vi "CreateEmptyExcelFile.vi"() -> ()   [LabVIEW 2013]
panel:
  in  "# Sheets":i32=1 min=1 step=1
  in  "sheetname":string="Sheet1"
  in  "File Name":path=path "C:/PhaeronGit/LVNPOI/Scratch/test.xls"
  # "LabVIEW implementation of CreateEmptyExcelFile.cs"
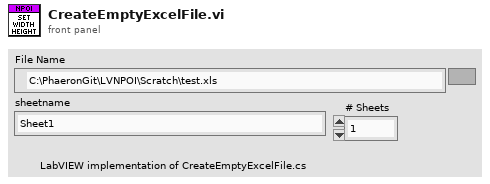
[diagram p1: front panel]
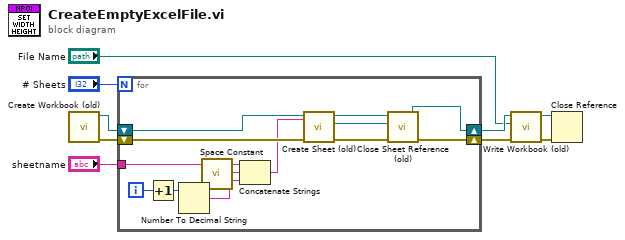
[diagram p0: block diagram]
diagram:
  n1 = call "Create Workbook (old).vi"() -> ("error out"=w8:errorcluster, "IWorkbook Reference"=w9:refnum<k24>)  [unwired: 10 in]
  n2 = for {
    N: "# Sheets" -> [_]
    shift-right: [w11] -> w6
    shift-left: w8 -> [w16]
    shift-right: [w13] -> w7
    shift-left: w9 -> [w14]
    tunnel: "sheetname" -> [w20]
    i -> [w21]
    n3 = Increment(x=w21) -> (x+1=w19:i32)
    n4 = Number To Decimal String(number=w19) -> (decimal integer string=w18:string)  [unwired: 1 in]
    n5 = call <vilib>:"Space Constant.vi"() -> ("String"=w17:string)
    n6 = Concatenate Strings(w20, w17, w18) -> (w15:string)
    n7 = call "Create Sheet (old).vi"("Sheet Name (Sheet1)"=w15, "error in (no error)"=w16, "IWorkbook Reference"=w14) -> ("error out"=w10:errorcluster, "Sheet Reference"=w12:refnum<k24>, "IWorkbook Reference out"=w13:refnum<k24>)  [unwired: 6 in]
    n8 = call "Close Sheet Reference (old).vi"("error in (no error)"=w10, "Sheet Reference"=w12) -> ("error out"=w11:errorcluster)  [unwired: 9 in]
  }
  n9 = call "Write Workbook (old).vi"("error in (no error)"=w6, "File Name"="File Name", "IWorkbook Reference"=w7) -> ("error out"=w3:errorcluster, "IWorkbook Reference Out"=w4:refnum<k24>)  [unwired: 7 in]
  n10 = Close Reference(reference=w4, error in (no error)=w3) -> ()  [unwired: 1 out]
